vi "WriteCustomError.vi"(1 "Message":string, 2 "Code":u32) -> (0 "error out":errorcluster)   [LabVIEW 2016]
doc: "Writes an \"error\" or to the driverstation. Useful for debugging."
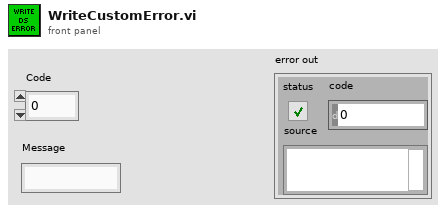
[diagram p1: front panel]
types:
  T1 = cluster{"Status":bool, "Code":u32, "Message":string}
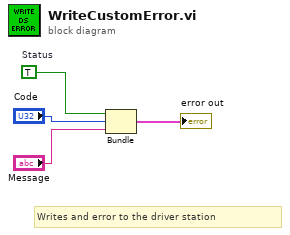
[diagram p0: block diagram]
diagram:
  w4 = TRUE  # Status
  # "Writes and error to the driver station"
  n1 = Bundle("Status"=w4, "Code"="Code", "Message"="Message") -> (→"error out":T1)  [unwired: 1 in]
